vi "Multiply Input Gain.vi"(8 "error in (no error)":errorcluster, 10 "WFM in":waveform(dbl)[](array[waveform]), 11 "Lockin.DAQ":refnum<class "Lockin.DAQ.lvclass">) -> (0 "error out":errorcluster, 2 "WFM out":waveform(dbl)[](array[waveform]), 3 "Lockin.DAQ out":refnum<class "Lockin.DAQ.lvclass">)   [LabVIEW 2016, in "Lockin.DAQ.lvclass"]
uses:
  Lockin.DAQ.lvclass
  Lockin.DAQ.lvclass/Lockin.DAQ.ctl
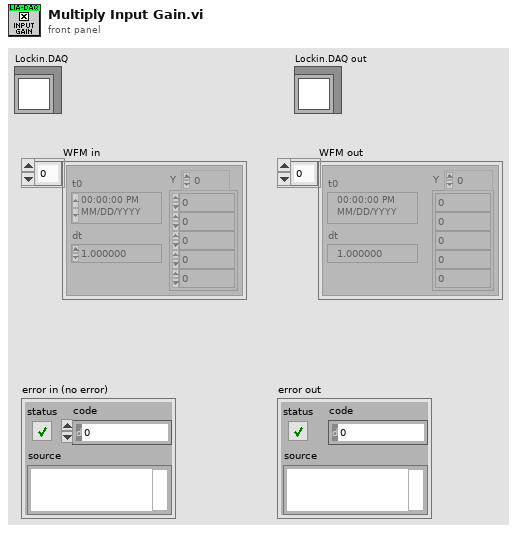
[diagram p1: front panel]
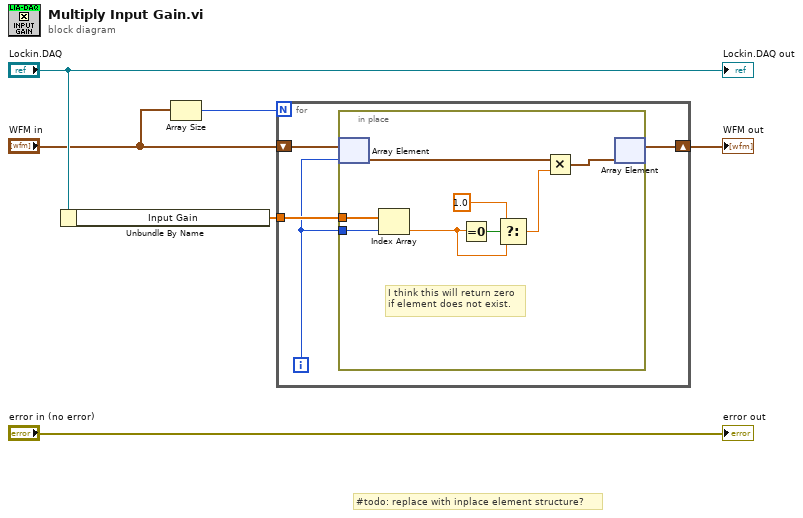
[diagram p0: block diagram]
diagram:
  # "#todo: replace with inplace element structure?"
  n1 = Unbundle By Name("Lockin.DAQ") -> ("Input Gain"=w3:dbl[])
  n2 = Array Size(array="WFM in") -> (size(s)=w1:i32)
  n3 = for {
    N: w1 -> [_]
    tunnel: w3 -> [w10]
    shift-right: [w9] -> w6
    shift-left: "WFM in" -> [w7]
    i -> [w8]
    n4 = in-place {
      in-place-border: w8 -> [w18]
      in-place-border: w10 -> [w17]
      # "I think this will return zero\nif element does not exist."
      n5 = in-place-array #1(w7, w8) -> (w12:waveform(dbl))
      n6 = Index Array(array=w17, index=w18) -> (element=w15:dbl)
      n7 = Equal To 0?(x=w15) -> (x = 0?=w16:bool)
      n8 = Select(t=1.0, s=w16, f=w15) -> (s? t:f=w14:dbl)
      n9 = Multiply(x=w12, y=w14) -> (x*y=w11:waveform(dbl))
      n10 = in-place-array #1(w11) -> (w9:waveform(dbl)[])  [unwired: 1 out]
    }
  }
  "WFM out" <- w6
  "error out" <- "error in (no error)"
  "Lockin.DAQ out" <- "Lockin.DAQ"
